vi "Untitled 2 (SubVI).vi"(10 "Passo":dbl=0.2, 11 "Faixa":dbl=2.0) -> (3 "Array":dbl[](array[numeric]))   [LabVIEW 2015]
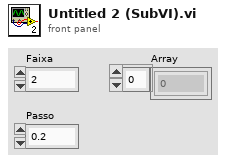
[diagram p1: front panel]
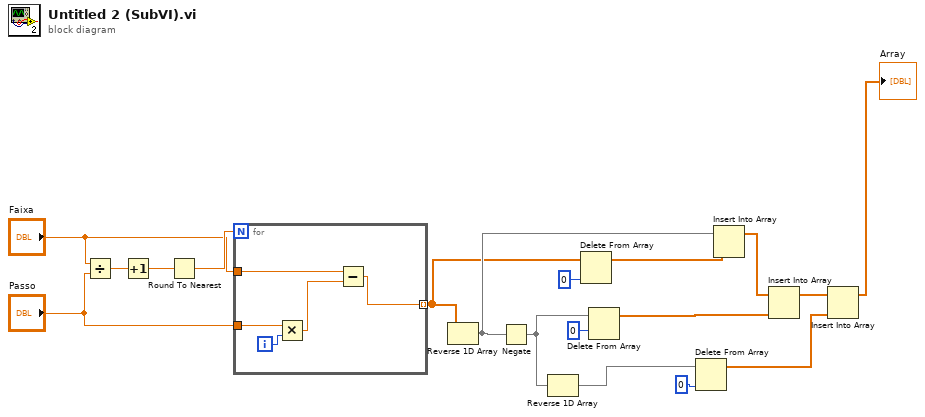
[diagram p0: block diagram]
diagram:
  n1 = Divide(x="Faixa", y="Passo") -> (x/y=w17:dbl)
  n2 = Increment(x=w17) -> (x+1=w3:dbl)
  n3 = Round To Nearest(number=w3) -> (nearest integer value=w16:dbl)
  n4 = for {
    N: w16 -> [_]
    tunnel: "Passo" -> [w22]
    tunnel: "Faixa" -> [w21]
    tunnel: [w19] -> w6 mode=indexing
    i -> [w23]
    n5 = Multiply(x=w22, y=w23) -> (x*y=w20:dbl)
    n6 = Subtract(x=w21, y=w20) -> (x-y=w19:dbl)
  }
  n7 = Reverse 1D Array(array=w6) -> (reversed array=w11:dbl[])
  n8 = Negate(x=w11) -> (-x=w8:dbl[])
  n9 = Reverse 1D Array(array=w8) -> (reversed array=w10:dbl[])
  n10 = Delete From Array(array=w6, index=0) -> (array with subset deleted=w12:dbl[])  [unwired: 1 in, 1 out]
  n11 = Delete From Array(array=w8, index=0) -> (array with subset deleted=w14:dbl[])  [unwired: 1 in, 1 out]
  n12 = Delete From Array(array=w10, index=0) -> (array with subset deleted=w2:dbl[])  [unwired: 1 in, 1 out]
  n13 = Insert Into Array(array=w11, new element=w12) -> (w13:dbl[])  [unwired: 1 in]
  n14 = Insert Into Array(array=w13, new element=w14) -> (w15:dbl[])  [unwired: 1 in]
  n15 = Insert Into Array(array=w15, new element=w2) -> (→"Array":dbl[])  [unwired: 1 in]
